vi "checkLongestSequence.vi"(8 "error in (no error)":errorcluster, 11 "Simon_Engine in":refnum<class "Simon_Engine.lvclass">) -> (0 "error out":errorcluster, 3 "Simon_Engine out":refnum<class "Simon_Engine.lvclass">)   [LabVIEW 2019, in "Simon_Engine.lvclass"]
uses:
  Simon_Engine.lvclass
  Simon_Engine.lvclass/Simon_Engine.ctl
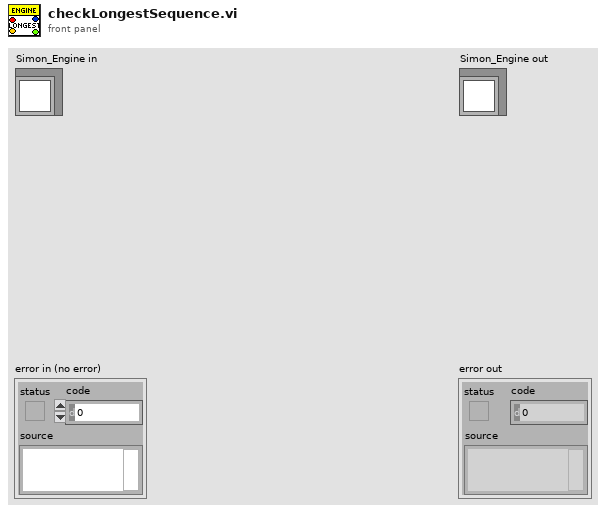
[diagram p1: front panel]
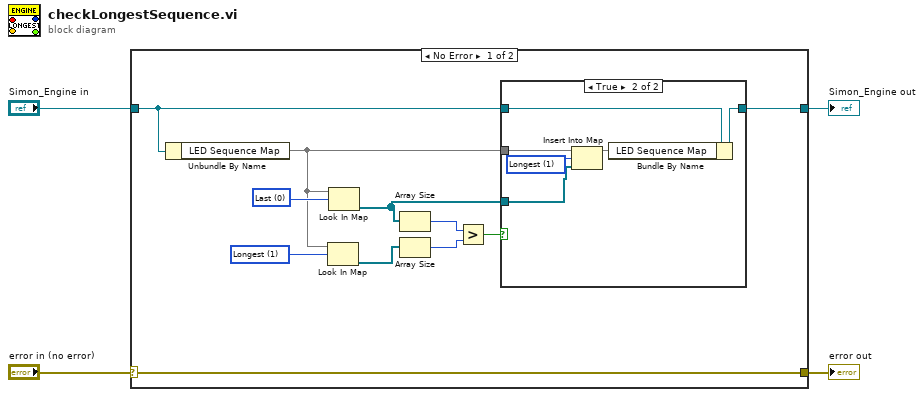
[diagram p0: block diagram]
diagram:
  n1 = case shown="No Error" "error in (no error)" {
    selector: "error in (no error)" -> [w15 w24]
    tunnel: [w15 w24] -> w3
    tunnel: [w13 w23] -> w1
    tunnel: "Simon_Engine in" -> [w14 w23]
    frame No Error {
      w11 = u8 1 items=["Last", "Longest"]
      w12 = u8 0 items=["Last", "Longest"]
      n2 = Unbundle By Name(w14) -> ("LED Sequence Map"=w7:map{u8, refnum<class "LED.lvclass">[]})
      n3 = Look In Map(map=w7, key=w11) -> (value=w8:refnum<class "LED.lvclass">[])  [unwired: 1 in, 1 out]
      n4 = Look In Map(map=w7, key=w12) -> (value=w5:refnum<class "LED.lvclass">[])  [unwired: 1 in, 1 out]
      n5 = Array Size(array=w5) -> (size(s)=w9:i32)
      n6 = Array Size(array=w8) -> (size(s)=w10:i32)
      n7 = Greater?(x=w9, y=w10) -> (0:w6:bool)
      n8 = case shown="True" w6 {
        tunnel: w14 -> [w16 w22]
        tunnel: [w16 w21] -> w13
        tunnel: w7 -> [_ w20]
        tunnel: w5 -> [_ w17]
        frame False {
        }
        frame True {
          w18 = u8 1 items=["Last", "Longest"]
          n9 = Insert Into Map(map in=w20, key=w18, value=w17) -> (map out=w19:map{u8, refnum<class "LED.lvclass">[]})  [unwired: 2 out]
          n10 = Bundle By Name(cluster=w22, "LED Sequence Map"=w19) -> (w21:refnum<class "Simon_Engine.lvclass">)
        }
      }
    }
    frame Error {
    }
  }
  "error out" <- w3
  "Simon_Engine out" <- w1
